vi "Register to Discovery Service.vi"(8 "error in":errorcluster, 10 "PortNumber":i32, 11 "gRPC ID":T2) -> (0 "error out":errorcluster, 2 "Response Data":T1, 3 "gRPC ID out":T2)   [LabVIEW 2020, in "CancellableMeasurement.lvlib"]
uses:
  CancellableMeasurement.lvlib
  <vilib>/gRPC/LabVIEW gRPC Library/Shared/grpcId.ctl
  <vilib>/MeasurementLink/Discovery Client/RPC Messages/ni_measurementlink_discovery_v1_RegisterServiceResponse.ctl
  <vilib>/MeasurementLink/Discovery Client/RPC Messages/ni_measurementlink_discovery_v1_RegisterServiceRequest.ctl
  <vilib>/MeasurementLink/Discovery Client/RPC Messages/ni_measurementlink_discovery_v1_ServiceDescriptor.ctl
  <vilib>/MeasurementLink/Discovery Client/RPC Messages/ni_measurementlink_discovery_v1_ServiceLocation.ctl
  <vilib>/MeasurementLink/Discovery Client/MeasurementLink Discovery Client.lvlib
  <vilib>/gRPC/LabVIEW gRPC Library/grpc-lvsupport-release.lvlib
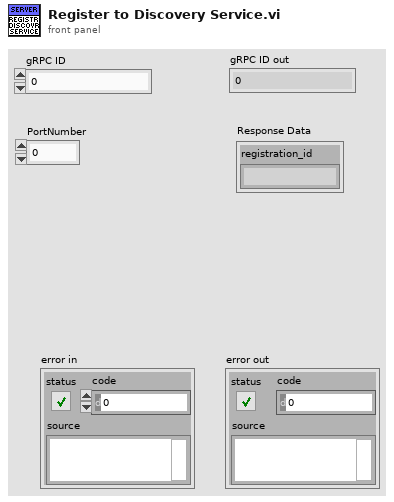
[diagram p1: front panel]
types:
  T1 = typedef "MeasurementLink Discovery Client.lvlib/ni_measurementlink_discovery_v1_RegisterServiceResponse.ctl" = cluster{"registration_id":string}
  T2 = typedef "grpc-lvsupport-release.lvlib/grpcId.ctl" = u64
  T3 = typedef "MeasurementLink Discovery Client.lvlib/ni_measurementlink_discovery_v1_RegisterServiceRequest.ctl" = cluster{"service_description":T4, "location":T5}
  T4 = typedef "MeasurementLink Discovery Client.lvlib/ni_measurementlink_discovery_v1_ServiceDescriptor.ctl" = cluster{"display_name":string, "description_url":string, "provided_interfaces":string[], "service_class":string}
  T5 = typedef "MeasurementLink Discovery Client.lvlib/ni_measurementlink_discovery_v1_ServiceLocation.ctl" = cluster{"location":string, "insecure_port":string, "ssl_authenticated_port":string}
  T6 = typedef "CancellableMeasurement.lvlib/ni_measurementlink_measurement_v1_MeasurementDetails.ctl" = cluster{"display_name":string, "version":string}
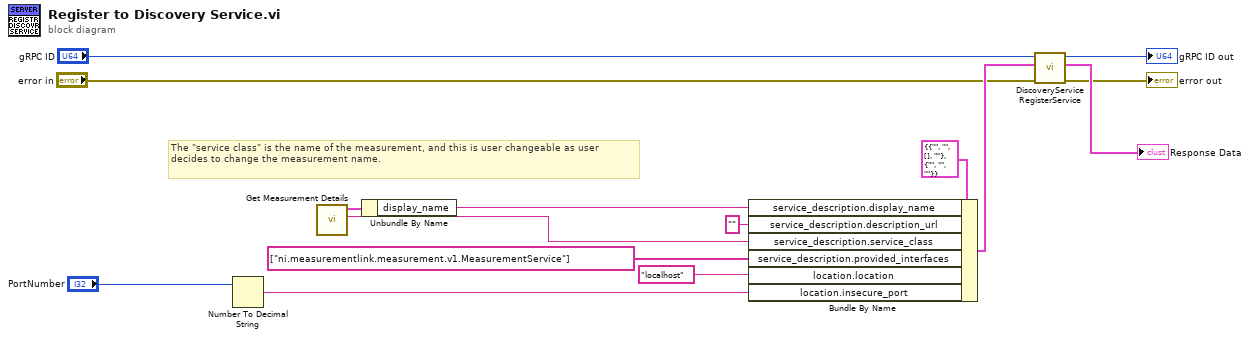
[diagram p0: block diagram]
diagram:
  # "The \"service class\" is the name of the measurement, and this is user changeable as user decides to change the measurement name."
  n1 = Number To Decimal String(number="PortNumber") -> (decimal integer string=w15:string)  [unwired: 1 in]
  n2 = call "Get Measurement Details.vi"() -> ("Service Class"=w8:string, "Measurement Details"=w13:T6)  [unwired: 9 in, 1 out]
  n3 = Unbundle By Name(w13) -> ("display_name"=w10:string)
  n4 = Bundle By Name(cluster=T3 {"service_description"={"display_name"="", "description_url"="", "provided_interfaces"=[], "service_class"=""}, "location"={"location"="", "insecure_port"="", "ssl_authenticated_port"=""}} ("Request Data"), "service_description.display_name"=w10, "service_description.description_url"="", "service_description.service_class"=w8, "service_description.provided_interfaces"=string[] ["ni.measurementlink.measurement.v1.MeasurementService"] ("provided_services"), "location.location"="localhost", "location.insecure_port"=w15) -> (w6:T3)
  n5 = call <vilib>:"DiscoveryService RegisterService.vi"("error in"="error in", "Request Data"=w6, "gRPC ID"="gRPC ID") -> ("error out"=→"error out":errorcluster, "Response Data"=→"Response Data":T1, "gRPC ID out"=→"gRPC ID out":T2)  [unwired: 6 in]
